vi "Actor Core.vi"(8 "error in":errorcluster, 11 "IED Status Logger in":refnum<class "IED Status Logger.lvclass">) -> (0 "error out":errorcluster, 3 "Actor out":refnum<class "Actor.lvclass">)   [LabVIEW 2018, in "IED Status Logger Actor.lvlib" / "IED Status Logger.lvclass"]
doc: "(<B>Filename</B>: Actor Framework.lvlib:Actor.lvclass:Actor Core.vi)\n\nReceives messages to the actor, reacts to them, and initiates any error handling that may shut the actor down.\n\nDescendant classes may override this VI to append parallel tasks for the actor to complete while it handles messages. Overrides use the Call Parent Method node."
uses:
  IED Status Logger.lvclass
  <vilib>/ActorFramework/Actor/Actor.lvclass
  IED Status Logger.lvclass/IED Status Logger.ctl
  <vilib>/ORNL/CSEISMIC DDS/CSEISMIC DDS Base/Data Types/IED_Status.ctl
  <vilib>/ORNL/CSEISMIC DDS/CSEISMIC DDS Base/Data Types/Controls/DeviceID.ctl
  <vilib>/ORNL/CSEISMIC DDS/CSEISMIC DDS Base/Data Types/Controls/Timestamp.ctl
  <vilib>/ORNL/CSEISMIC DDS/CSEISMIC DDS Base/CSEISMIC DDS.lvclass
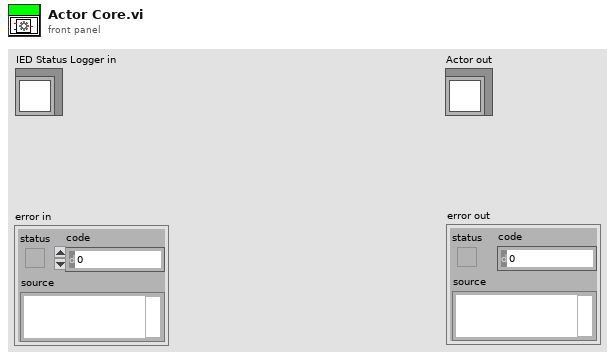
[diagram p1: front panel]
types:
  T1 = enum16{"open", "open or create", "create or replace", "create", "open (read-only)"}
  T2 = typedef "EMS Generic Actor.lvlib/EMS Generic.lvclass/Data Type DVRs.ctl" = cluster{"IED_Status":refnum<data-value>, "IED_Status_0":refnum<data-value>, "DER_Measurement":refnum<data-value>, "DER_Info":refnum<data-value>, "DER_Status":refnum<data-value>, "ES_Measurement":refnum<data-value>, "ES_Info":refnum<data-value>, "PV_Info":refnum<data-value>, "SmartRelay_Info":refnum<data-value>, "SmartRelay_Measurement":refnum<data-value>, "Meter_Info":refnum<data-value>, "Meter_Measurement":refnum<data-value>, "HVAC_Status":refnum<data-value>, "HVAC_Measurement":refnum<data-value>, "PriceData_RealTime":refnum<data-value>, "PriceData_Demand":refnum<data-value>, "PriceData_Energy":refnum<data-value>, "ForecastData_Long":refnum<data-value>, "ForecastData_Short":refnum<data-value>, "DER_Control":refnum<data-value>, "DER_SetPointF":refnum<data-value>, "DER_SetPointP":refnum<data-value>, "DER_SetPointQ":refnum<data-value>, "DER_SetPointPF":refnum<data-value>, "DER_SetPointV":refnum<data-value>, "PV_setCurtailment":refnum<data-value>, "PV_setRampRate":refnum<data-value>, "Relay_Control":refnum<data-value>, "Load_Control":refnum<data-value>, "HVAC_Control":refnum<data-value>, "Generator_Info":refnum<data-value>, "ForecastData_Long_Backup":refnum<data-value>, "PriceData_RealTime_Backup":refnum<data-value>}
  T3 = typedef "CSEISMIC DDS.lvlib/CSEISMIC DDS.lvclass/IED_Status.ctl" = cluster{"DeviceID":T4, "Timestamp":T5, "MicrogridID":u8, "Active":bool, "Inactive":bool, "Error":i32, "Fault":bool, "ErrorString":string}
  T4 = typedef "CSEISMIC DDS.lvlib/CSEISMIC DDS.lvclass/DeviceID.ctl" = string
  T5 = typedef "CSEISMIC DDS.lvlib/CSEISMIC DDS.lvclass/Timestamp.ctl" = cluster{"Seconds":u64, "Remainder":u64}
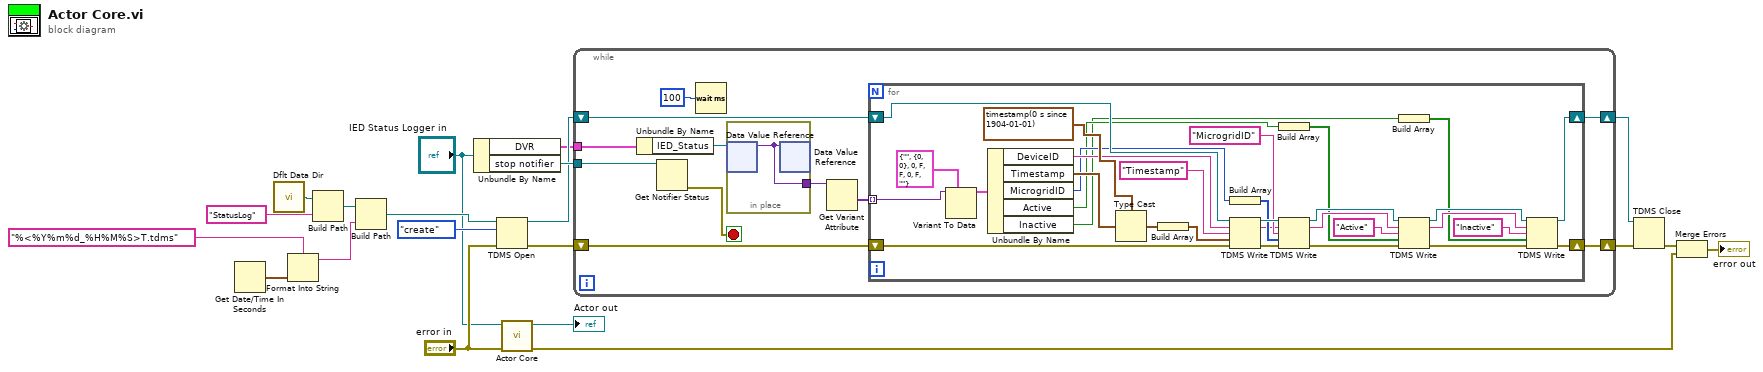
[diagram p0: block diagram]
diagram:
  n1 = Get Date/Time In Seconds() -> (seconds since 1Jan1904=w15:timestamp)
  n2 = call <vilib>:"Dflt Data Dir.vi"() -> ("App:Default Data Directory"=w18:path)
  n3 = Format Into String(format string="%<%Y%m%d_%H%M%S>T.tdms", w15) -> (resulting string=w13:string)  [unwired: 2 in, 1 out]
  n4 = Build Path(base path=w18, name or relative path="StatusLog") -> (appended path=w16:path)
  n5 = Build Path(base path=w16, name or relative path=w13) -> (appended path=w12:path)
  n6 = Unbundle By Name("IED Status Logger in") -> ("DVR"=w5:T2, "stop notifier"=w9:refnum<notifier>)
  n7 = TDMS Open(8:"error in", 10:T1."create" ("operation (0:open)"), 11:w12) -> (0:w7:errorcluster, 3:w8:refnum<k34>)  [unwired: 4 in]
  n8 = call-parent "Actor Core.vi"("error in"="error in", "Actor in"="IED Status Logger in") -> ("error out"=w20:errorcluster, "Actor out"=→"Actor out":refnum<class "Actor.lvclass">)  [unwired: 8 in]
  n9 = while {
    tunnel: w9 -> [w31]
    shift-right: [w23] -> w4
    shift-left: w8 -> [w26]
    shift-right: [w22] -> w3
    shift-left: w7 -> [w25]
    tunnel: w5 -> [w29]
    stop <- w30 stop-if-true
    n10 = Unbundle By Name(w29) -> ("IED_Status"=w28:refnum<data-value>)
    n11 = Get Notifier Status(notifier=w31) -> (error out=w30:errorcluster)  [unwired: 1 in, 4 out]
    n12 = Wait (ms)(milliseconds to wait=u32 100) -> ()  [unwired: 1 out]
    n13 = in-place {
      in-place-border: [w63] -> w27
      n14 = in-place-dvr #1(w28) -> (w63:variant)  [unwired: 1 out]
      n15 = in-place-dvr #1(w63) -> ()  [unwired: 2 out]
    }
    n16 = Get Variant Attribute(Variant=w27) -> (values=w24:variant[])  [unwired: 3 in, 3 out]
    n17 = for {
      shift-right: [w33] -> w23
      shift-left: w26 -> [w62]
      shift-right: [w32] -> w22
      shift-left: w25 -> [w61]
      tunnel: w24 -> [w60] mode=indexing
      n18 = Variant To Data(type=T3 {"DeviceID"="", "Timestamp"={"Seconds"=0, "Remainder"=0}, "MicrogridID"=0, "Active"=FALSE, "Inactive"=FALSE, "Error"=0, "Fault"=FALSE, "ErrorString"=""} ("IED_Status"), Variant=w60) -> (data=w58:T3)  [unwired: 1 in, 1 out]
      n19 = Unbundle By Name(w58) -> ("DeviceID"=w52:T4, "Timestamp"=w57:T5, "MicrogridID"=w48:u8, "Active"=w41:bool, "Inactive"=w35:bool)
      n20 = Type Cast(type=timestamp(0 s since 1904-01-01), x=w57) -> (*(type *) &x=w54:timestamp)
      n21 = Build Array(w54) -> (w53:timestamp[])
      n22 = Build Array(w48) -> (w47:u8[])
      n23 = TDMS Write(0:w62, 5:w52, 7:"Timestamp" ("String"), 9:w53, 11:w61) -> (4:w50:refnum<k34>, 6:w43:string, 15:w51:errorcluster)  [unwired: 1 in, 1 out]
      n24 = Build Array(w41) -> (w40:bool[])
      n25 = TDMS Write(0:w50, 5:w43, 7:"MicrogridID" ("String"), 9:w47, 11:w51) -> (4:w46:refnum<k34>, 6:w44:string, 15:w45:errorcluster)  [unwired: 1 in, 1 out]
      n26 = Build Array(w35) -> (w34:bool[])
      n27 = TDMS Write(0:w46, 5:w44, 7:"Active" ("String"), 9:w40, 11:w45) -> (4:w38:refnum<k34>, 6:w37:string, 15:w36:errorcluster)  [unwired: 1 in, 1 out]
      n28 = TDMS Write(0:w38, 5:w37, 7:"Inactive" ("String"), 9:w34, 11:w36) -> (4:w33:refnum<k34>, 15:w32:errorcluster)  [unwired: 1 in, 2 out]
    }
  }
  n29 = TDMS Close(8:w3, 11:w4) -> (0:w1:errorcluster)  [unwired: 1 out]
  n30 = Merge Errors(w1, w20) -> (→"error out":errorcluster)
